vi "搜索文件和进度条.vi"() -> ()   [LabVIEW 2023]
panel:
  out "进度条":dbl(slide) scale=0.0..1.0
  out "文件总数":i32
  out "VI 文件":string[](array[string])
  in  "Path":path
  # "在一个指定文件夹里列出所有VI文件 并且 显示 完成搜索进度"
  # "/Users/yuxintong/Labview-examples"
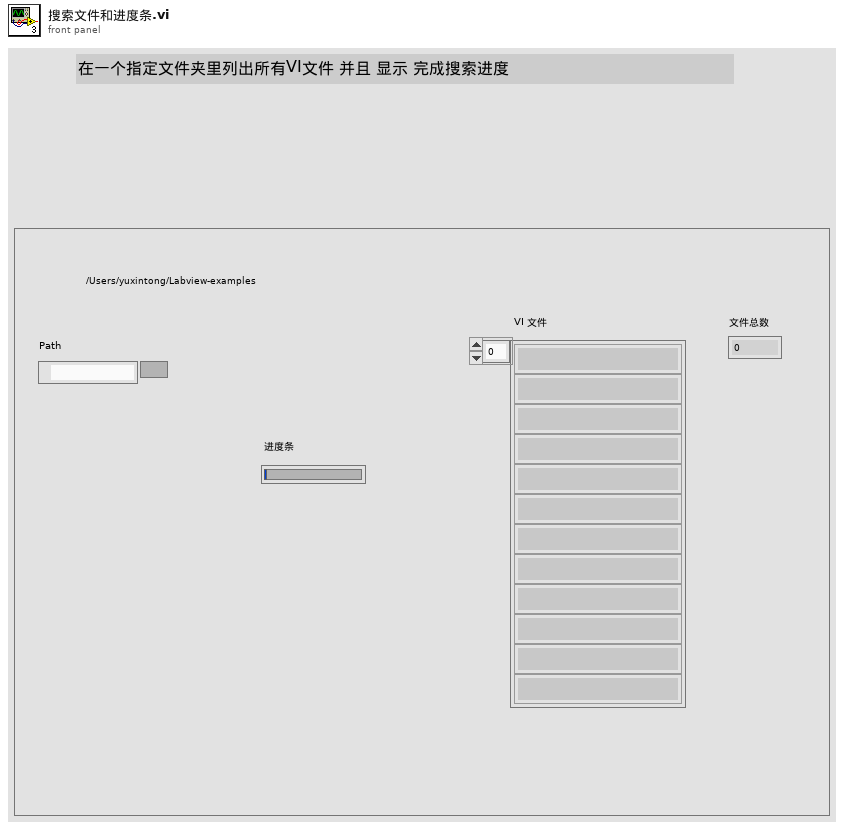
[diagram p1: front panel]
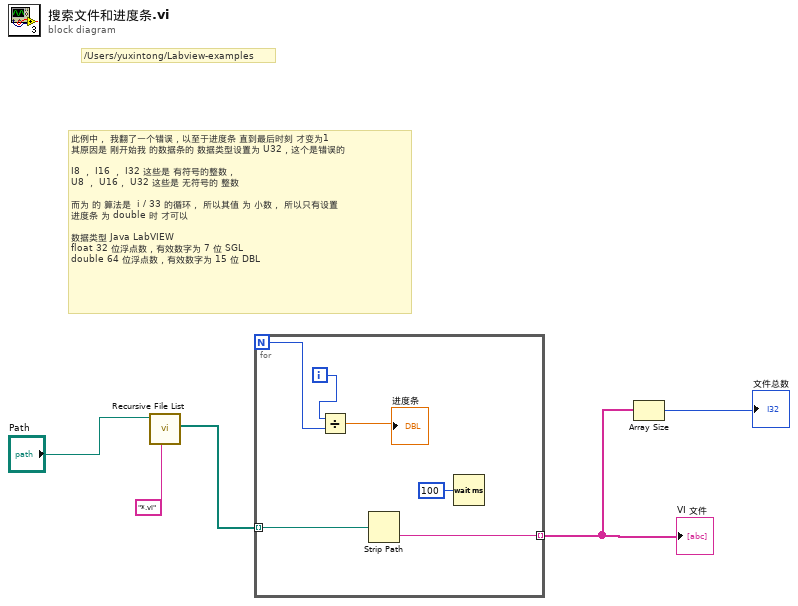
[diagram p0: block diagram]
diagram:
  # "/Users/yuxintong/Labview-examples"
  # "此例中， 我翻了一个错误，以至于进度条 直到最后时刻 才变为1 \n其原因是 刚开始我 的数据条的 数据类型设置为 U32，这个是错误的\n\nI8 ， I16 ， I32 这些是 有符号的整数， \nU8 ， U16， U32 这些是 无符号的 整数\n\n而为 的 算法是  i / 33 的循环， 所以其值 为 小数， 所以只有设置\n进度条 为 double 时 才可以\n\n数据类型\tJava\tLabVIEW\nfloat\t32 位浮点数，有效数字为 7 位\tSGL\ndouble\t64 位浮点数，有效数字为 15 位\tDBL"
  n1 = call <vilib>:"Recursive File List.vi"("pattern"="*.vi", "Folder Path"="Path") -> ("All Files in Dir"=w3:path[])  [unwired: 5 in, 4 out]
  n2 = for {
    N -> [w9]
    tunnel: w3 -> [w11] mode=indexing
    tunnel: [w10] -> w1 mode=indexing
    i -> [w6]
    n3 = Divide(x=w6, y=w9) -> (x/y=→"进度条":dbl)
    n4 = Strip Path(path=w11) -> (name=w10:string)  [unwired: 1 out]
    n5 = Wait (ms)(milliseconds to wait=u32 100) -> ()  [unwired: 1 out]
  }
  "VI 文件" <- w1
  n6 = Array Size(array=w1) -> (size(s)=→"文件总数":i32)
